vi "Part 2.vi"(11 "Input":string) -> (3 "Output":i32)   [LabVIEW 2021]
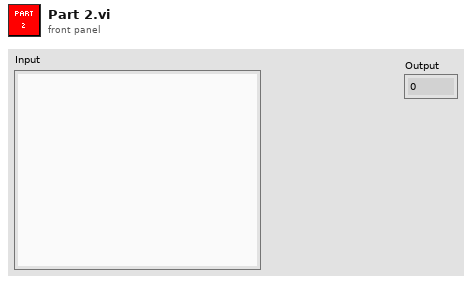
[diagram p1: front panel]
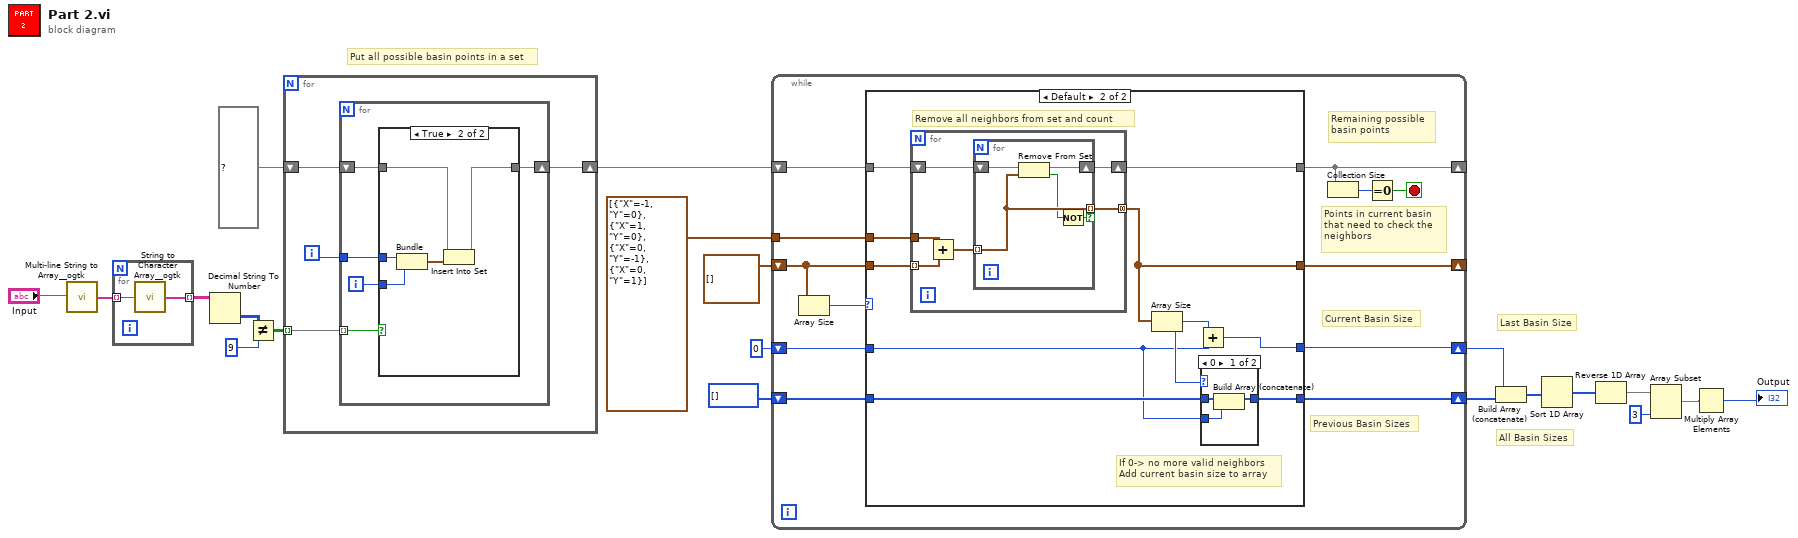
[diagram p0: block diagram]
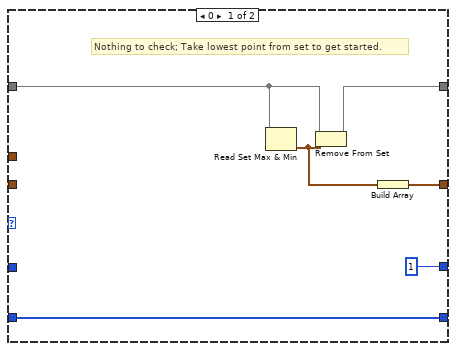
[diagram p3: hidden frame]
diagram:
  # "All Basin Sizes"
  # "Last Basin Size"
  # "Put all possible basin points in a set"
  n1 = call <userlib>:"Multi-line String to Array__ogtk.vi"("string"="Input") -> ("lines"=w20:string[])
  n2 = for {
    tunnel: w20 -> [w22] mode=indexing
    tunnel: [w21] -> w19 mode=indexing
    n3 = call <userlib>:"String to Character Array__ogtk.vi"("Input String"=w22) -> ("Character Array"=w21:string[])
  }
  n4 = Decimal String To Number(string=w19) -> (number=w17:i32[][])  [unwired: 2 in, 1 out]
  n5 = Not Equal?(x=w17, y=9) -> (x != y?=w14:bool[][])
  n6 = for {
    tunnel: w14 -> [w25] mode=indexing
    shift-right: [w24] -> w12
    shift-left: set{cluster{"X":i32, "Y":i32}} {} ("set in") -> [w26]
    i -> [w23]
    n7 = for {
      shift-right: [w30] -> w24
      shift-left: w26 -> [w31]
      tunnel: w25 -> [w29] mode=indexing
      tunnel: w23 -> [w27]
      i -> [w28]
      n8 = case shown="True" w29 {
        tunnel: w31 -> [w32 w37]
        tunnel: [w32 w36] -> w30
        tunnel: w28 -> [_ w35]
        tunnel: w27 -> [_ w34]
        frame False {
        }
        frame True {
          n9 = Bundle(w34, w35) -> (w33:cluster{i32, i32})  [unwired: 1 in]
          n10 = Insert Into Set(10:w33, 11:w37) -> (3:w36:set{cluster{"X":i32, "Y":i32}})  [unwired: 1 out]
        }
      }
    }
  }
  n11 = while {
    shift-right: [w45] -> _
    shift-left: w12 -> [w46]
    shift-right: [w43] -> _
    shift-left: cluster{"X":i32, "Y":i32}[] [] ("appended array") -> [w40]
    shift-right: [w44] -> w7
    shift-left: 0 -> [w38]
    shift-right: [w41] -> w8
    shift-left: i32[] [] -> [w42]
    tunnel: cluster{"X":i32, "Y":i32}[] [{"X"=-1, "Y"=0}, {"X"=1, "Y"=0}, {"X"=0, "Y"=-1}, {"X"=0, "Y"=1}] -> [w39]
    stop <- w48 stop-if-true
    # "Remaining possible\nbasin points"
    # "Points in current basin\nthat need to check the \nneighbors"
    # "Previous Basin Sizes"
    # "Current Basin Size"
    n12 = Array Size(array=w40) -> (size(s)=w47:i32)
    n13 = case shown="Default" w47 {
      tunnel: w46 -> [w54 w63]
      tunnel: [w55 w62] -> w45
      tunnel: [1 w60] -> w44
      tunnel: [w52 w61] -> w43
      tunnel: w42 -> [w50 w58]
      tunnel: [w50 w57] -> w41
      tunnel: w40 -> [_ w65]
      tunnel: w39 -> [_ w64]
      tunnel: w38 -> [_ w56]
      frame 0 {
        # "Nothing to check; Take lowest point from set to get started."
        n14 = Read Set Max & Min(11:w54) -> (1:w51:cluster{"X":i32, "Y":i32})  [unwired: 1 out]
        n15 = Remove From Set(10:w51, 11:w54) -> (3:w55:set{cluster{"X":i32, "Y":i32}})  [unwired: 1 out]
        n16 = Build Array(w51) -> (w52:cluster{"X":i32, "Y":i32}[])
      }
      frame Default {
        # "If 0-> no more valid neighbors\nAdd current basin size to array"
        # "Remove all neighbors from set and count"
        n17 = for {
          tunnel: w65 -> [w75] mode=indexing
          tunnel: w64 -> [w74]
          shift-right: [w72] -> w62
          shift-left: w63 -> [w73]
          tunnel: [w70] -> w61 mode=concatenating
          n18 = Add(x=w74, y=w75) -> (x+y=w71:cluster{"X":i32, "Y":i32}[])
          n19 = for {
            tunnel: w71 -> [w78] mode=indexing
            shift-right: [w79] -> w72
            shift-left: w73 -> [w80]
            tunnel: [w78] -> w70 mode=indexing if=w76
            n20 = Remove From Set(10:w78, 11:w80) -> (2:w77:bool, 3:w79:set{cluster{"X":i32, "Y":i32}})
            n21 = Not(x=w77) -> (.not. x?=w76:bool)
          }
        }
        n22 = Array Size(array=w61) -> (size(s)=w59:i32)
        n23 = Add(x=w59, y=w56) -> (x+y=w60:i32)
        n24 = case shown="0" w59 {
          tunnel: w58 -> [w68 w69]
          tunnel: [w66 w69] -> w57
          tunnel: w56 -> [w67 _]
          frame 0 {
            n25 = Build Array (concatenate)(w68, w67) -> (w66:i32[])
          }
          frame Default {
          }
        }
      }
    }
    n26 = Collection Size(1:w45) -> (0:w49:i32)
    n27 = Equal To 0?(x=w49) -> (x = 0?=w48:bool)
  }
  n28 = Build Array (concatenate)(w7, w8) -> (w6:i32[])
  n29 = Sort 1D Array(array=w6) -> (sorted array=w5:i32[])
  n30 = Reverse 1D Array(array=w5) -> (reversed array=w4:i32[])
  n31 = Array Subset(array=w4, length=3) -> (w2:i32[])  [unwired: 1 in]
  n32 = Multiply Array Elements(1:w2) -> (0:→"Output":i32)
